vi "PointerToArrayEX.vi"(0 "Array in":u8[](array[numeric]), 1 "Pointer In":u64, 2 "Pointer Size":u64, 3 "error in (no error)":errorcluster) -> (7 "Array out":u8[](array[numeric]), 9 "error out":errorcluster)   [LabVIEW 2019]
doc: "Pointer To Array\n\nOutput:\n U8[] Array out \n\nInput:\n U8[] Array in\n U64 Pointer in\n\nPopulates an array from its pointer."
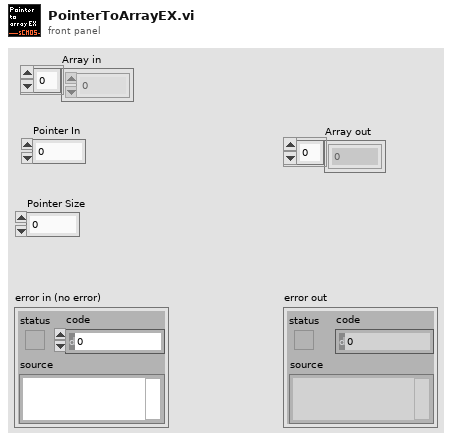
[diagram p1: front panel]
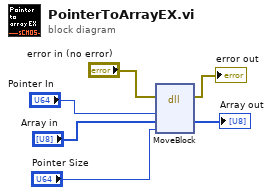
[diagram p0: block diagram]
diagram:
  n1 = dll-call lib="LabVIEW" fn="MoveBlock"(error in="error in (no error)", "Address (Pointer)"="Pointer In", "Destination"="Array in", "Size"="Pointer Size") -> (error out=→"error out":errorcluster, "Destination"=→"Array out":u8[])  [unwired: 5 in, 1 out]
